vi "Config dialog.vi"(8 "error in (no error)":errorcluster, 10 "Camera config in":T2={"Camera session"="Webcam", "VideoMode"=0}, 11 "Arduino config in":T3) -> (0 "error out":errorcluster, 1 "Cancelled?":bool, 2 "Camera config out":T2, 3 "Arduino config out":T3)   [LabVIEW 2020]
uses:
  controls/Arduino config -- cluster.ctl
  controls/Camera config parameters -- cluster.ctl
  <vilib>/userdefined/High Color/IMAQdx.ctl
  controls/Config dialog states.ctl
  Camera/Libraries/Camera/Connection type--enum.ctl
  <vilib>/vision/driver/NI_Vision_Acquisition_Software.lvlib
  Camera/Libraries/Camera/Camera.lvlib
panel:
  in  "VISA resource":refnum<visa-resource-name> caption="Arduino port"
  in  "Video modes":u32(ring) items=["Max 1216x1936"]
  in  "Camera session":T1
  out "Camera config (old)":T2
  out "Arduino config (old)":T3
  in  "Cancel Button":bool
  in  "OK Button":bool
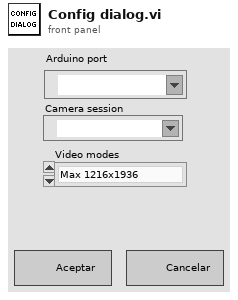
[diagram p1: front panel]
types:
  T1 = typedef "IMAQdx.ctl" = refnum<k21>
  T2 = typedef "Camera config parameters -- cluster.ctl" = cluster{"Camera session":T1, "VideoMode":u32}
  T3 = typedef "Arduino config -- cluster.ctl" = cluster{"VISA resource":refnum<visa-resource-name>}
  T4 = typedef "Config dialog states.ctl" = enum16{"Initialize", "Wait", "Exit"}
  T5 = typedef "Camera.lvlib/Connection type--enum.ctl" = enum16{"GigE", "USB", "Simulated"}
  T6 = cluster{"Video Mode":u32, "Video Mode Name":string}[]
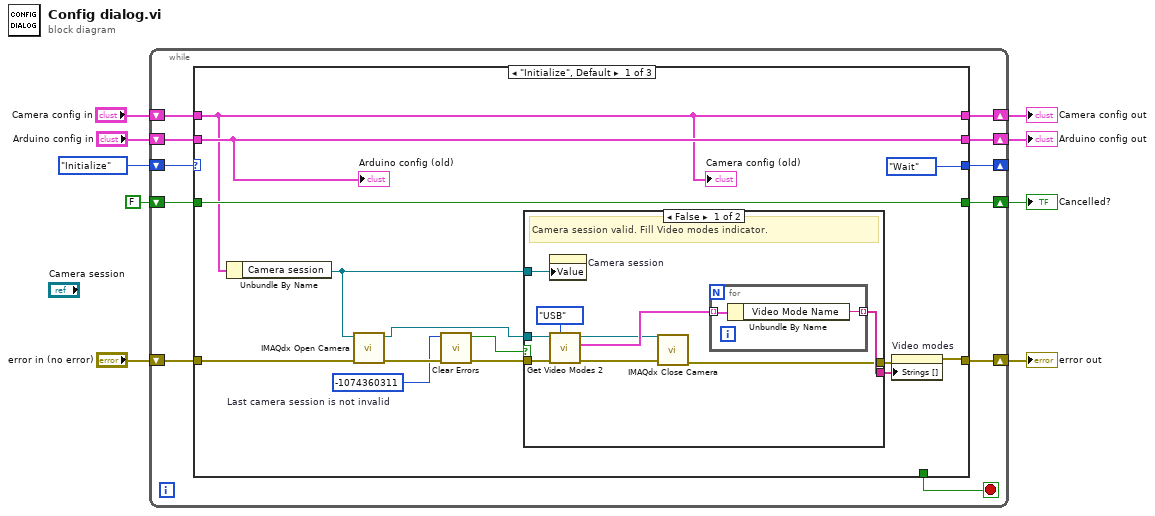
[diagram p0: block diagram]
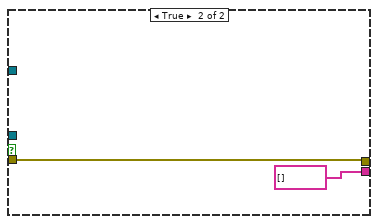
[diagram p2: hidden frame]
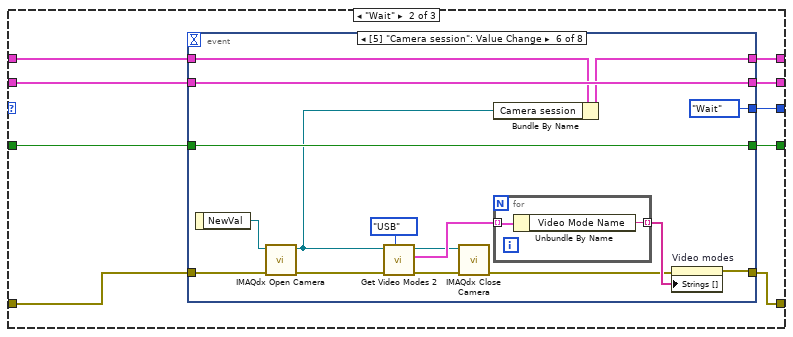
[diagram p3: hidden frame]
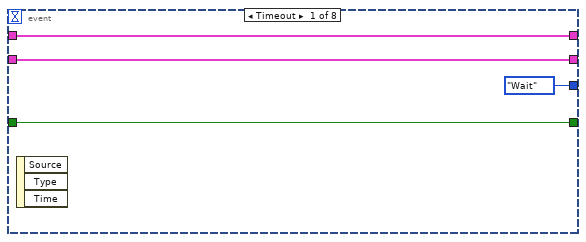
[diagram p4: hidden frame]
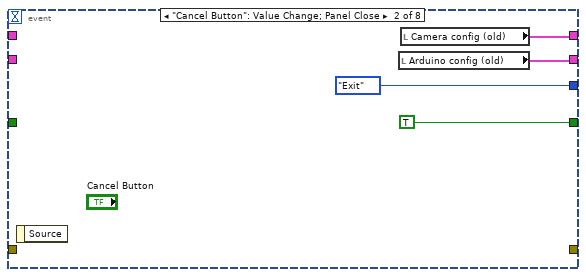
[diagram p5: hidden frame]
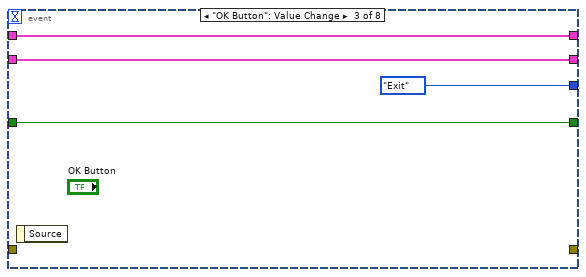
[diagram p6: hidden frame]
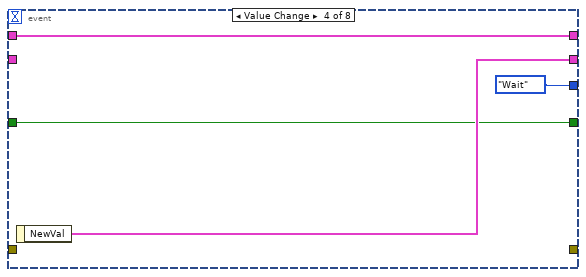
[diagram p7: hidden frame]
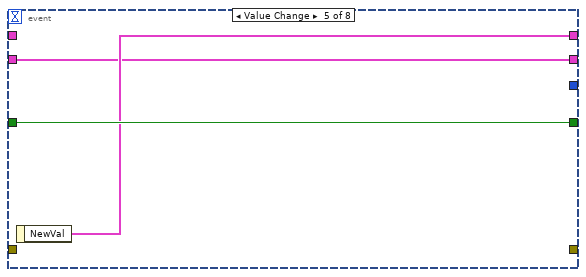
[diagram p8: hidden frame]
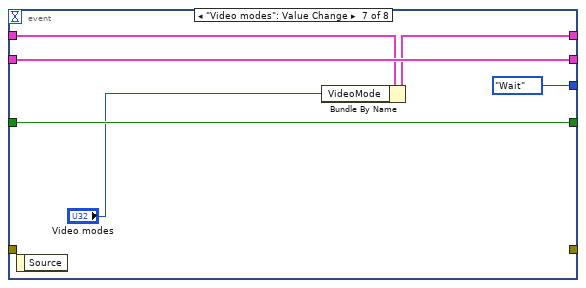
[diagram p9: hidden frame]
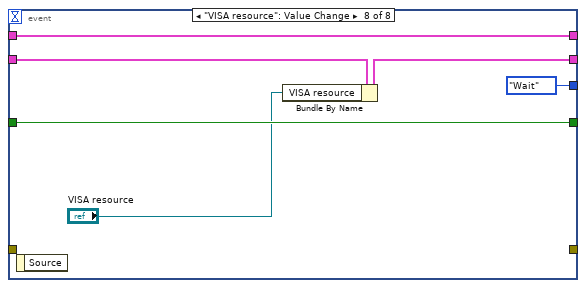
[diagram p10: hidden frame]
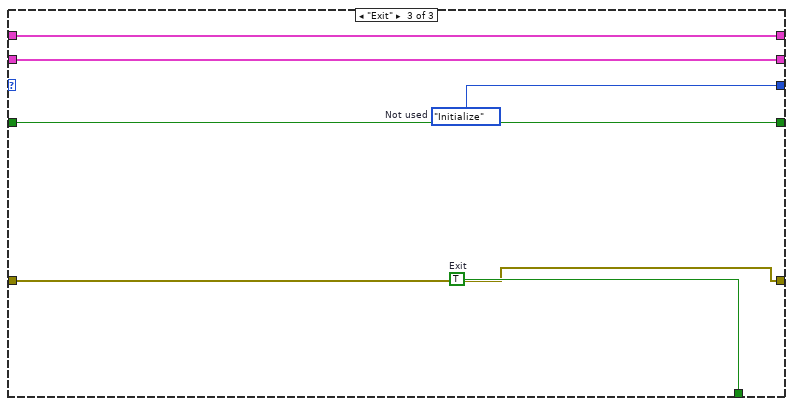
[diagram p11: hidden frame]
diagram:
  n1 = while {
    shift-right: [w18] -> _
    shift-left: Config_dialog_states."Initialize" -> [w20]
    shift-right: [w16] -> w7
    shift-left: "error in (no error)" -> [w17]
    shift-right: [w14] -> w5
    shift-left: "Arduino config in" -> [w15]
    shift-right: [w13] -> w4
    shift-left: FALSE -> [w12]
    shift-right: [w10] -> w1
    shift-left: "Camera config in" -> [w11]
    stop <- w19 stop-if-true
    n2 = case shown="\"Initialize\", Default" w20 {
      tunnel: [_ _ w111] -> w19
      tunnel: [Config_dialog_states."Wait" w54 w108] -> w18
      tunnel: w17 -> [w26 w49 w110]
      tunnel: [w31 w48 w110] -> w16
      tunnel: w15 -> [w33 w56 w109]
      tunnel: [w33 w55 w109] -> w14
      tunnel: [w32 w53 w107] -> w13
      tunnel: w12 -> [w32 w52 w107]
      tunnel: w11 -> [w29 w50 w106]
      tunnel: [w29 w51 w106] -> w10
      frame "Initialize", Default {
        w22 = -1074360311  # Last camera session is not invalid
        n3 = Unbundle By Name(w29) -> ("Camera session"=w28:T1)
        n4 = call <vilib>:"IMAQdx Open Camera.vi"("error in"=w26, "Session In"=w28) -> ("error out"=w25:errorcluster, "Session Out"=w24:T1)  [unwired: 8 in]
        n5 = call <vilib>:"Clear Errors.vi"("error in (no error)"=w25, "specific error code to clear (0: all)"=w22) -> ("error out"=w23:errorcluster, "specific error cleared?"=w21:bool)  [unwired: 4 in]
        n6 = case shown="False" w21 {
          tunnel: [w43 string[] []] -> w30
          tunnel: w28 -> [w42 _]
          tunnel: [w41 w47] -> w27
          tunnel: w24 -> [w37 _]
          tunnel: w23 -> [w35 w47]
          frame False {
            # "Camera session valid. Fill Video modes indicator."
            n7 = property on="Camera session" class="IMAQdx (strict)"("Value"=w42) -> ()  [unwired: 2 in, 2 out]
            n8 = call "Get Video Modes 2.vi"("Connection type"=Connection_type--enum."USB", "error in (no error)"=w35, "Cam session in"=w37) -> ("error out"=w39:errorcluster, "Video modes"=w38:T6, "Cam session out"=w36:T1)  [unwired: 5 in, 1 out]
            n9 = call <vilib>:"IMAQdx Close Camera.vi"("error in"=w39, "Session In"=w36) -> ("error out"=w41:errorcluster)  [unwired: 9 in]
            n10 = for {
              tunnel: w38 -> [w45] mode=indexing
              tunnel: [w44] -> w43 mode=indexing
              n11 = Unbundle By Name(w45) -> ("Video Mode Name"=w44:string)
            }
          }
          frame True {
          }
        }
        n12 = property on="Video modes" class="Ring (strict)"(error in=w27, "Strings []"=w30) -> (error out=w31:errorcluster)  [unwired: 1 in, 1 out]
        "Arduino config (old)" <- w33
        "Camera config (old)" <- w29
      }
      frame "Wait" {
        n13 = event shown="[5] \"Camera session\": Value Change" {
          selector: _ -> [_ _ _ _ _ _ _ _]
          dyn-events: _ -> [_ _ _ _ _ _ _ _]
          timeout: _ -> [_ _ _ _ _ _ _ _]
          tunnel: w56 -> [w60 _ w68 _ w73 w88 w98 w103]
          tunnel: [w60 w64 w68 w72 w73 w88 w98 w101] -> w55
          tunnel: [Config_dialog_states."Wait" Config_dialog_states."Exit" Config_dialog_states."Exit" Config_dialog_states."Wait" _ Config_dialog_states."Wait" Config_dialog_states."Wait" Config_dialog_states."Wait"] -> w54
          tunnel: [w58 TRUE w66 w70 w75 w91 w99 w105] -> w53
          tunnel: w52 -> [w58 _ w66 w70 w75 w91 w99 w105]
          tunnel: [w57 w61 w65 w69 w74 w86 w95 w104] -> w51
          tunnel: w50 -> [w57 _ w65 w69 _ w87 w97 w104]
          tunnel: w49 -> [_ _ _ _ _ w84 _ _]
          tunnel: [_ _ _ _ _ w89 _ _] -> w48
          event Timeout {
            n14 = event-data() -> ()  [unwired: 1 in, 3 out]
          }
          event "Cancel Button": Value Change; Panel Close {
            n15 = event-data() -> ()  [unwired: 1 in, 1 out]
            n16 = local read "Arduino config (old)"() -> (w64:T3)
            n17 = local read "Camera config (old)"() -> (w61:T2)
          }
          event "OK Button": Value Change {
            n18 = event-data() -> ()  [unwired: 1 in, 1 out]
          }
          event Value Change {
            n19 = event-data() -> ("NewVal"=w72:T3)  [unwired: 1 in]
          }
          event Value Change {
            n20 = event-data() -> ("NewVal"=w74:T2)  [unwired: 1 in]
          }
          event Value Change {
            n21 = event-data() -> ("NewVal"=w82:T1)  [unwired: 1 in]
            n22 = call <vilib>:"IMAQdx Open Camera.vi"("error in"=w84, "Session In"=w82) -> ("error out"=w81:errorcluster, "Session Out"=w79:T1)  [unwired: 8 in]
            n23 = call "Get Video Modes 2.vi"("Connection type"=Connection_type--enum."USB", "error in (no error)"=w81, "Cam session in"=w79) -> ("error out"=w77:errorcluster, "Video modes"=w80:T6, "Cam session out"=w78:T1)  [unwired: 5 in, 1 out]
            n24 = call <vilib>:"IMAQdx Close Camera.vi"("error in"=w77, "Session In"=w78) -> ("error out"=w83:errorcluster)  [unwired: 9 in]
            n25 = Bundle By Name(cluster=w87, "Camera session"=w79) -> (w86:T2)
            n26 = for {
              tunnel: w80 -> [w93] mode=indexing
              tunnel: [w92] -> w90 mode=indexing
              n27 = Unbundle By Name(w93) -> ("Video Mode Name"=w92:string)
            }
            n28 = property on="Video modes" class="Ring (strict)"(error in=w83, "Strings []"=w90) -> (error out=w89:errorcluster)  [unwired: 1 in, 1 out]
          }
          event "Video modes": Value Change {
            n29 = event-data() -> ()  [unwired: 1 in, 1 out]
            n30 = Bundle By Name(cluster=w97, "VideoMode"="Video modes") -> (w95:T2)
          }
          event "VISA resource": Value Change {
            n31 = event-data() -> ()  [unwired: 1 in, 1 out]
            n32 = Bundle By Name(cluster=w103, "VISA resource"="VISA resource") -> (w101:T3)
          }
        }
      }
      frame "Exit" {
        w108 = Config_dialog_states."Initialize"  # Not used
        w111 = TRUE  # Exit
      }
    }
  }
  "error out" <- w7
  "Arduino config out" <- w5
  "Cancelled?" <- w4
  "Camera config out" <- w1
